vi "move_which_direction.vi"(10 "MOVE TO POSITION":i32, 11 "Current Valve":i32) -> (3 "Move Clockwise?":bool)   [LabVIEW 2013]
panel:
  out "CCW MOVES":i32
  out "CW MOVES":i32
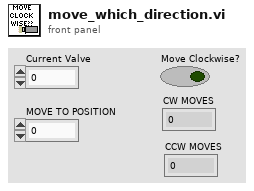
[diagram p1: front panel]
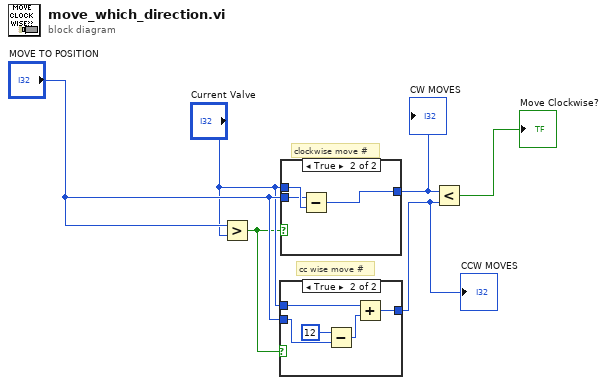
[diagram p0: block diagram]
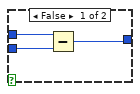
[diagram p2: hidden frame]
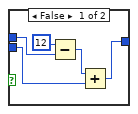
[diagram p3: hidden frame]
diagram:
  # "cc wise move #"
  # "clockwise move #"
  n1 = Greater?(x="MOVE TO POSITION", y="Current Valve") -> (0:w1:bool)
  n2 = case shown="True" w1 {
    tunnel: [w7 w10] -> w5
    tunnel: "Current Valve" -> [w9 w12]
    tunnel: "MOVE TO POSITION" -> [w8 w13]
    frame False {
      n3 = Subtract(x=w9, y=w8) -> (x-y=w7:i32)
    }
    frame True {
      n4 = Subtract(x=12, y=w13) -> (x-y=w11:i32)
      n5 = Add(x=w12, y=w11) -> (x+y=w10:i32)
    }
  }
  "CCW MOVES" <- w5
  n6 = case shown="True" w1 {
    tunnel: "Current Valve" -> [w17 w21]
    tunnel: "MOVE TO POSITION" -> [w19 w20]
    tunnel: [w15 w22] -> w4
    frame False {
      n7 = Subtract(x=12, y=w17) -> (x-y=w16:i32)
      n8 = Add(x=w16, y=w19) -> (x+y=w15:i32)
    }
    frame True {
      n9 = Subtract(x=w20, y=w21) -> (x-y=w22:i32)
    }
  }
  "CW MOVES" <- w4
  n10 = Less?(x=w4, y=w5) -> (x < y?=→"Move Clockwise?":bool)
